vi "Find Instrument Addon Custom Device.vi"(8 "error in":errorcluster, 11 "target in":refnum<k24>) -> (0 "error out":errorcluster, 1 "NodeID":u64, 3 "target out":refnum<k24>)   [LabVIEW 2019]
uses:
  NationalInstruments.VeriStand.SystemDefinitionAPI
  <vilib>/NI VeriStand/Custom Device API/Custom Device Item Ref.ctl
  <vilib>/NI VeriStand/Custom Device API/Custom Device API.lvlib
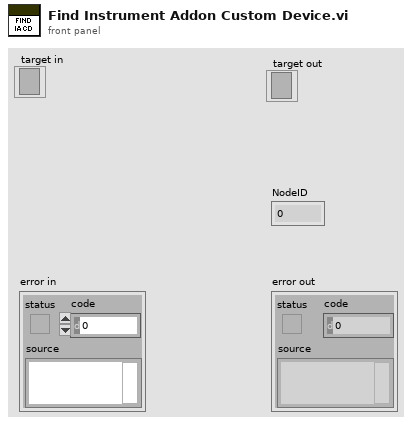
[diagram p1: front panel]
types:
  T1 = typedef "Custom Device API.lvlib/Custom Device Item Ref.ctl" = u64
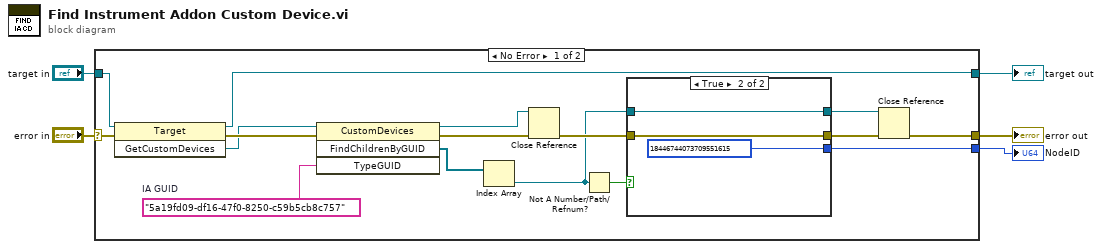
[diagram p0: block diagram]
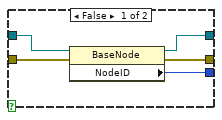
[diagram p2: hidden frame]
diagram:
  n1 = case shown="No Error" "error in" {
    selector: "error in" -> [w21 w31]
    tunnel: [w10 w31] -> w5
    tunnel: "target in" -> [w20 w30]
    tunnel: [w14 w30] -> w2
    tunnel: [w12 _] -> w1
    frame No Error {
      w6 = "5a19fd09-df16-47f0-8250-c59b5cb8c757"  # IA GUID
      n2 = invoke class="Target" method="GetCustomDevices"(reference=w20, error in=w21) -> (reference out=w14:refnum<k24>, error out=w19:errorcluster, "GetCustomDevices"=w18:refnum<k24>)  [unwired: 1 in]
      n3 = invoke class="CustomDevices" method="FindChildrenByGUID"(reference=w18, error in=w19, "TypeGUID"=w6) -> (reference out=w17:refnum<k24>, error out=w16:errorcluster, "FindChildrenByGUID"=w8:refnum<k24>[])  [unwired: 1 in, 1 out]
      n4 = Index Array(array=w8) -> (element=w7:refnum<k24>)  [unwired: 1 in]
      n5 = Close Reference(reference=w17, error in (no error)=w16) -> (error out=w15:errorcluster)
      n6 = Not A Number/Path/Refnum?(number/path/refnum=w7) -> (NaN/Path/Refnum?=w13:bool)
      n7 = case shown="True" w13 {
        tunnel: [w22 w29] -> w9
        tunnel: w15 -> [w24 w29]
        tunnel: w7 -> [w26 w28]
        tunnel: [w25 T1 18446744073709551615 ("command refnum")] -> w12
        tunnel: [w23 w28] -> w11
        frame False {
          n8 = property class="BaseNode"(reference=w26, error in=w24) -> (reference out=w23:refnum<k24>, error out=w22:errorcluster, "NodeID"=w25:u64)
        }
        frame True {
        }
      }
      n9 = Close Reference(reference=w11, error in (no error)=w9) -> (error out=w10:errorcluster)
    }
    frame Error {
    }
  }
  "target out" <- w2
  "error out" <- w5
  "NodeID" <- w1
